vi "subWriteBuildOrderToLogFile.vi"(8 "error in (no error)":errorcluster, 11 "SolutionBuilder in":refnum<class "SolutionBuilder.lvclass">) -> (0 "error out":errorcluster, 3 "SolutionBuilder out":refnum<class "SolutionBuilder.lvclass">)   [LabVIEW 2019, in "SolutionBuilder.lvlib" / "SolutionBuilder.lvclass"]
uses:
  SolutionBuilder.lvclass
  SolutionBuilder.lvclass/SolutionBuilder.ctl
  ProjectItem/ProjectItem.lvclass
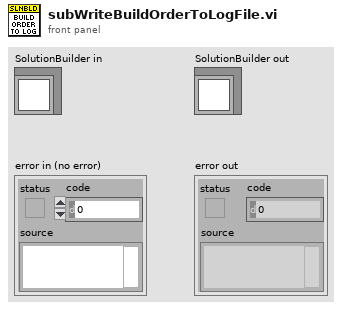
[diagram p1: front panel]
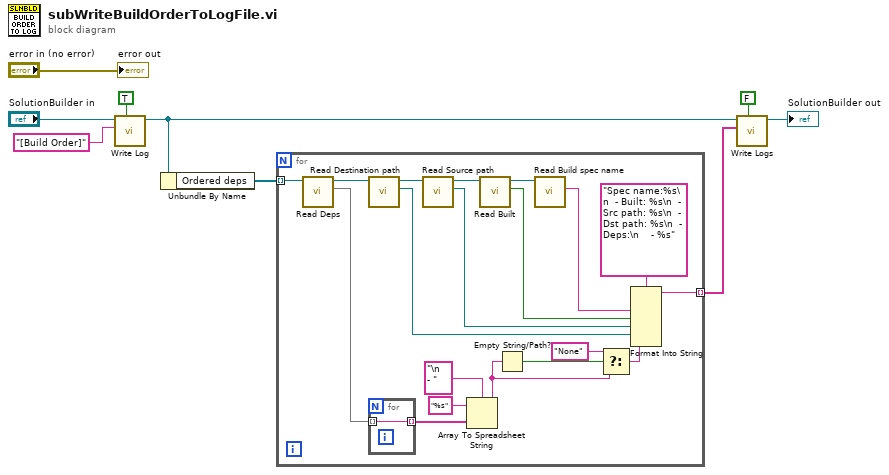
[diagram p0: block diagram]
diagram:
  n1 = call "Write Log.vi"("Prepend timestamp"=TRUE, "Log entry"="[Build Order]", "SolutionBuilder in"="SolutionBuilder in") -> ("SolutionBuilder out"=w3:refnum<class "SolutionBuilder.lvclass">)  [unwired: 8 in]
  n2 = Unbundle By Name(w3) -> ("Ordered deps"=w5:refnum<class "ProjectItem.lvclass">[])
  n3 = for {
    tunnel: w5 -> [w28] mode=indexing
    tunnel: [w18] -> w4 mode=indexing
    n4 = call "Read Deps.vi"("ProjectItem in"=w28) -> ("Deps"=w17:set{string}, "ProjectItem out"=w27:refnum<class "ProjectItem.lvclass">)  [unwired: 9 in]
    n5 = call "Read Destination path.vi"("ProjectItem in"=w27) -> ("Destination path"=w20:path, "ProjectItem out"=w26:refnum<class "ProjectItem.lvclass">)  [unwired: 9 in]
    n6 = for {
      tunnel: w17 -> [w29] mode=indexing
      tunnel: [w29] -> w16 mode=indexing
    }
    n7 = call "Read Source path.vi"("ProjectItem in"=w26) -> ("Source path"=w21:path, "ProjectItem out"=w25:refnum<class "ProjectItem.lvclass">)  [unwired: 9 in]
    n8 = Array To Spreadsheet String(delimiter (Tab)="\n    - ", array=w16, 3:"%s" ("format string")) -> (spreadsheet string=w10:string)
    n9 = call "Read Built.vi"("ProjectItem in"=w25) -> ("Built"=w22:bool, "ProjectItem out"=w24:refnum<class "ProjectItem.lvclass">)  [unwired: 9 in]
    n10 = Empty String/Path?(string/path=w10) -> (empty?=w13:bool)
    n11 = call "Read Build spec name.vi"("ProjectItem in"=w24) -> ("Build spec name"=w23:string)  [unwired: 9 in, 1 out]
    n12 = Select(t="None" ("format string"), s=w13, f=w10) -> (s? t:f=w11:string)
    n13 = Format Into String(format string="Spec name:%s\n  - Built: %s\n  - Src path: %s\n  - Dst path: %s\n  - Deps:\n    - %s", w23, w22, w21, w20, w11) -> (resulting string=w18:string)  [unwired: 2 in, 1 out]
  }
  n14 = call "Write Logs.vi"("Prepend timestamp"=FALSE, "Log entries"=w4, "SolutionBuilder in"=w3) -> ("SolutionBuilder out"=→"SolutionBuilder out":refnum<class "SolutionBuilder.lvclass">)  [unwired: 8 in]
  "error out" <- "error in (no error)"
